vi "multiplierA.vi"(1 "Integration Period (s)":dbl, 4 "Input":T1 {"Input Signal" format="%.2f"; "LOCK-IN Freq" format="%.2f"; "LOCK-IN Phase" format="%.2f"; "Time Constant (sec)" format="%.2f"; "Low-pass filter scope" format="%.2f"; "Time" format="%.2f"; "Spectral Amplitude" format="%.2f"; "Phase Angle" format="%.2f"; "Frequency" format="%.2f"; "Amplitude" format="%.2f"}) -> (0 "OUTPUT":T2 {"Input Signal" format="%.2f"; "Ch 2 Mult" format="%.2f"; "Ch 1 Mult" format="%.2f"; "LOCK-IN Freq" format="%.2f"; "LOCK-IN Phase" format="%.2f"; "Time Constant (sec)" format="%.2f"; "Low-pass filter slope" format="%.2f"; "Time" format="%.2f"; "Noise Amplitude" format="%.2f"; "Phase Angle" format="%.2f"; "Frequency" format="%.2f"; "Amplitude" format="%.2f"}, 2 "ymod":dbl[](array[numeric]), 3 "xmod":dbl[](array[numeric]))   [LabVIEW 2013]
doc: "Performs the Lock-In's integration / mixing by multiplying the input signal by the reference signal."
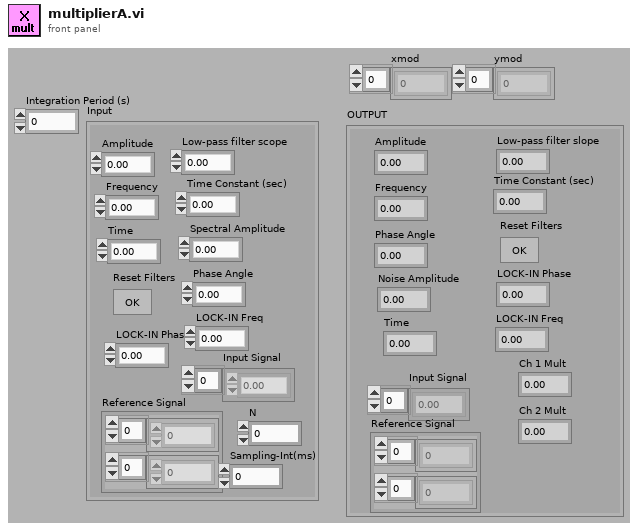
[diagram p1: front panel]
types:
  T1 = cluster{"Amplitude":dbl, "Frequency":dbl, "Phase Angle":dbl, "Spectral Amplitude":dbl, "Time":dbl, "Low-pass filter scope":dbl, "Time Constant (sec)":dbl, "Reset Filters":bool, "LOCK-IN Phase":dbl, "LOCK-IN Freq":dbl, "Sampling-Int(ms)":dbl, "Reference Signal":cluster{dbl[], dbl[]}, "Input Signal":dbl[], "N":i32}
  T2 = cluster{"Amplitude":dbl, "Frequency":dbl, "Phase Angle":dbl, "Noise Amplitude":dbl, "Time":dbl, "Low-pass filter slope":dbl, "Time Constant (sec)":dbl, "Reset Filters":bool, "LOCK-IN Phase":dbl, "LOCK-IN Freq":dbl, "Input Signal":dbl[], "Ch 1 Mult":dbl, "Ch 2 Mult":dbl, "Reference Signal":cluster{dbl[], dbl[]}}
  T3 = cluster{"Amplitude":dbl, "Frequency":dbl, "Phase Angle":dbl, "Spectral Amplitude":dbl, "Time":dbl, "Low-pass filter scope":dbl, "Time Constant (sec)":dbl, "Reset Filters":bool, "LOCK-IN Phase":dbl, "LOCK-IN Freq":dbl, "Input Signal":dbl[], dbl, dbl, cluster{dbl[], dbl[]}}
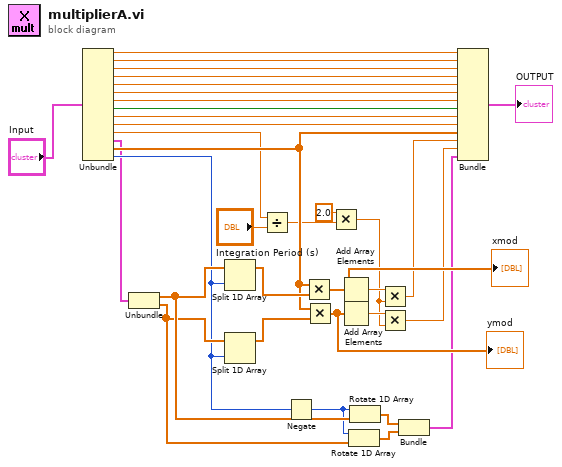
[diagram p0: block diagram]
diagram:
  n1 = Unbundle("Input") -> ("Amplitude"=w34:dbl, "Frequency"=w12:dbl, "Phase Angle"=w33:dbl, "Spectral Amplitude"=w32:dbl, "Time"=w31:dbl, "Low-pass filter scope"=w30:dbl, "Time Constant (sec)"=w29:dbl, "Reset Filters"=w28:bool, "LOCK-IN Phase"=w27:dbl, "LOCK-IN Freq"=w25:dbl, "Sampling-Int(ms)"=w8:dbl, "Reference Signal"=w2:cluster{dbl[], dbl[]}, "Input Signal"=w11:dbl[], "N"=w4:i32)
  n2 = Unbundle(w2) -> (w20:dbl[], w17:dbl[])
  n3 = Split 1D Array(array=w20, index=w4) -> (first subarray=w19:dbl[])  [unwired: 1 out]
  n4 = Split 1D Array(array=w17, index=w4) -> (first subarray=w18:dbl[])  [unwired: 1 out]
  n5 = Divide(x=w8, y="Integration Period (s)") -> (x/y=w5:dbl)
  n6 = Negate(x=w4) -> (-x=w10:i32)
  n7 = Multiply(x=w11, y=w19) -> (x*y=w24:dbl[])
  "xmod" <- w24
  n8 = Multiply(x=w11, y=w18) -> (x*y=w3:dbl[])
  "ymod" <- w3
  n9 = Multiply(x=2.0, y=w5) -> (x*y=w6:dbl)
  n10 = Add Array Elements(numeric array=w24) -> (sum=w14:dbl)
  n11 = Add Array Elements(numeric array=w3) -> (sum=w16:dbl)
  n12 = Rotate 1D Array(1:w17, 2:w10) -> (0:w21:dbl[])
  n13 = Rotate 1D Array(1:w20, 2:w10) -> (0:w22:dbl[])
  n14 = Multiply(x=w14, y=w6) -> (x*y=w13:dbl)
  n15 = Multiply(x=w16, y=w6) -> (x*y=w15:dbl)
  n16 = Bundle(w22, w21) -> (w1:cluster{dbl[], dbl[]})  [unwired: 1 in]
  n17 = Bundle("Amplitude"=w34, "Frequency"=w12, "Phase Angle"=w33, "Spectral Amplitude"=w32, "Time"=w31, "Low-pass filter scope"=w30, "Time Constant (sec)"=w29, "Reset Filters"=w28, "LOCK-IN Phase"=w27, "LOCK-IN Freq"=w25, "Input Signal"=w11, w13, w15, w1) -> (→"OUTPUT":T3)  [unwired: 1 in]
